vi "Remote Stream Control.vi"(9 "empty":bool, 10 "data valid":bool, 11 "stream.state in":T1) -> (1 "ready for start":bool, 2 "send data":bool, 3 "stream.state":T1, 4 "force requests":bool)   [LabVIEW 2015, in "niInstr Streaming v1 FPGA.lvlib"]
uses:
  <instrlib>/_niInstr/Streaming/v1/FPGA/niInstr Streaming v1 FPGA.lvlib
  <instrlib>/_niInstr/Streaming/v1/Common/Stream State.ctl
  <instrlib>/_niInstr/Streaming/v1/Common/niInstr Streaming v1 Common.lvlib
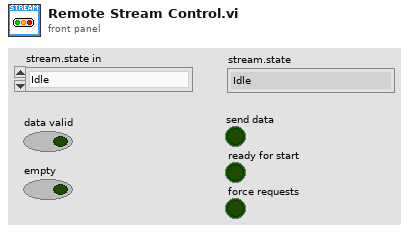
[diagram p1: front panel]
types:
  T1 = typedef "niInstr Streaming v1 Common.lvlib/Stream State.ctl" = enum8{"Idle", "Finite Transfer", "Continuous", "Done", "Error", "Not Ready", "Cancel"}
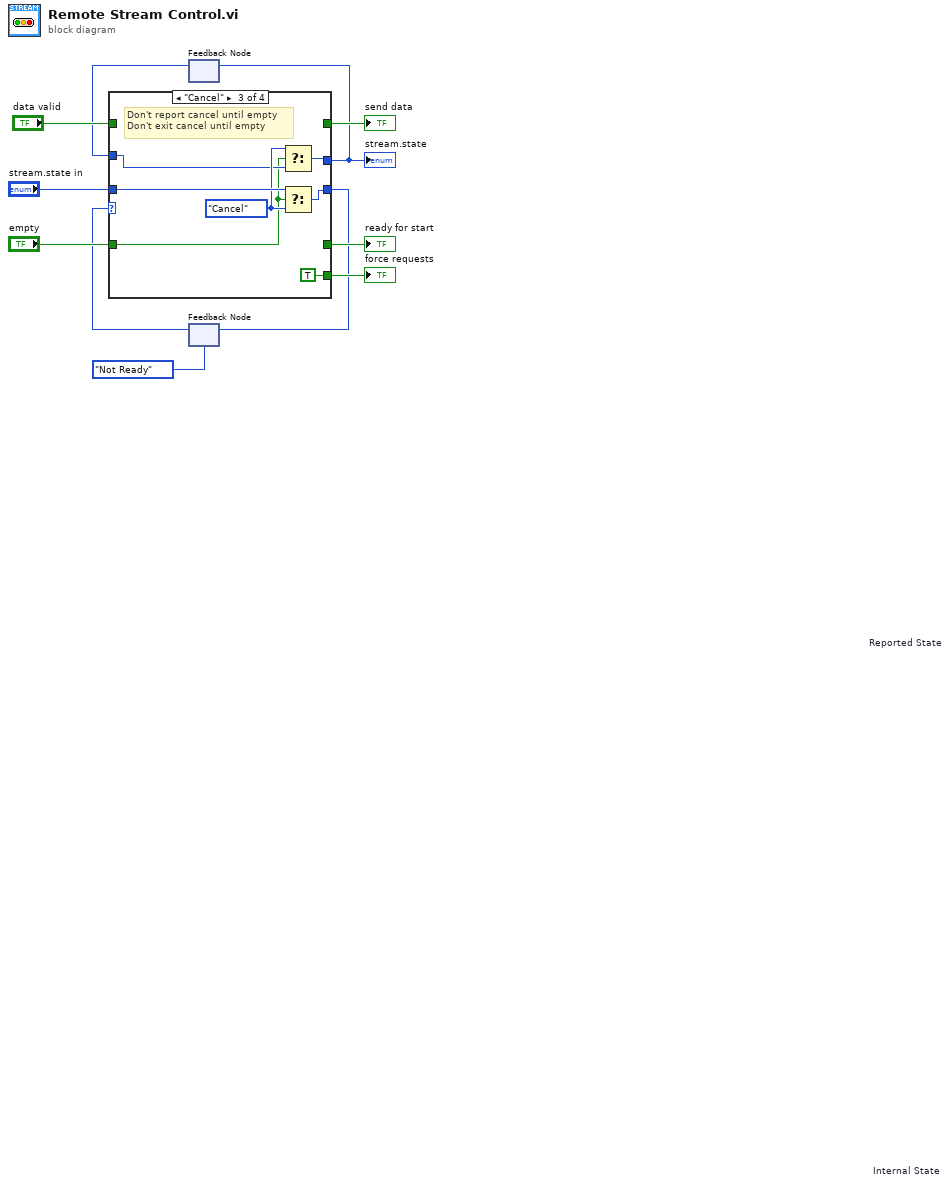
[diagram p0: block diagram]
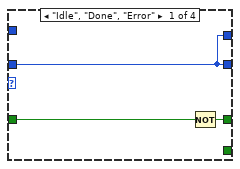
[diagram p2: hidden frame]
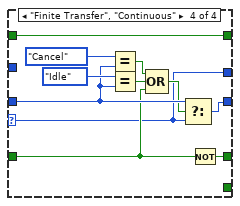
[diagram p4: hidden frame]
diagram:
  n1 = feedback #1 "Reported State"() -> (w2:T1)  [unwired: 1 in]
  n2 = feedback #2 "Internal State"(Stream_State."Not Ready" ("stream.state 0")) -> (w9:T1)
  n3 = case shown="\"Cancel\"" w9 {
    selector: w9 -> [_ _ _ w23]
    tunnel: "empty" -> [w14 _ w16 w25]
    tunnel: [w13 _ _ w33] -> w6
    tunnel: "stream.state in" -> [w12 w15 w21 w30]
    tunnel: [w12 w15 w20 w24] -> w1
    tunnel: [_ _ TRUE _] -> w10
    tunnel: "data valid" -> [_ _ _ w32]
    tunnel: [_ _ _ w32] -> w4
    tunnel: [w12 w15 w19 w23] -> w3
    tunnel: w2 -> [_ _ w17 _]
    frame "Idle", "Done", "Error" {
      n4 = Not(x=w14) -> (.not. x?=w13:bool)
    }
    frame "Not Ready" {
    }
    frame "Cancel" {
      w18 = Stream_State."Cancel" ("stream.state 0")
      # "Don't report cancel until empty\nDon't exit cancel until empty"
      n5 = Select(t=w18, s=w16, f=w17) -> (s? t:f=w19:T1)
      n6 = Select(t=w21, s=w16, f=w18) -> (s? t:f=w20:T1)
    }
    frame "Finite Transfer", "Continuous" {
      n7 = Equal?(x=Stream_State."Cancel" ("stream.state n"), y=w30) -> (x = y?=w27:bool)
      n8 = Equal?(x=Stream_State."Idle" ("stream.state n"), y=w30) -> (x = y?=w28:bool)
      n9 = Compound Arithmetic op=OR(w27, w28, w25) -> (w26:bool)
      n10 = Select(t=w30, s=w26, f=w23) -> (s? t:f=w24:T1)
      n11 = Not(x=w25) -> (.not. x?=w33:bool)
    }
  }
  "force requests" <- w10
  "stream.state" <- w3
  "ready for start" <- w6
  "send data" <- w4
  n12 = feedback-in #1(w3) -> ()
  n13 = feedback-in #2(w1) -> ()
